vi "Delete Device.vi"(8 "Error In":errorcluster, 11 "Device In":T1) -> (0 "error out":errorcluster)   [LabVIEW 2012]
doc: "Deletes an OpenCLV device."
uses:
  Non-User VIs/Controls/Device ID.ctl
  Non-User VIs/Buffers/Buffer_states.ctl
  OpenCLV x64.lvlib
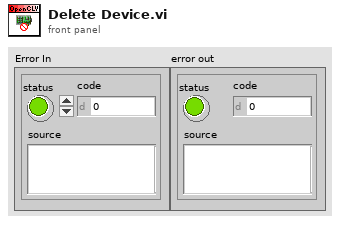
[diagram p1: front panel]
types:
  T1 = typedef "OpenCLV x64.lvlib/Device ID.ctl" = u64
  T2 = typedef "OpenCLV x64.lvlib/Buffer_states.ctl" = enum16{"Purge", "Remove", "Add"}
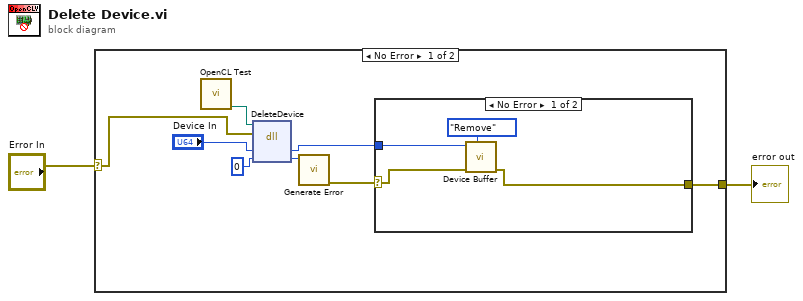
[diagram p0: block diagram]
diagram:
  n1 = case shown="No Error" "Error In" {
    selector: "Error In" -> [w3 w16]
    tunnel: [w10 w16] -> w2
    frame No Error {
      n2 = call "OpenCL Test.vi"() -> ("DLL To Use"=w4:path)  [unwired: 11 in]
      n3 = dll-call lib="C:/Users/bme-amcelroy-la/Desktop/OpenCLV/trunk/OpenCLV_x64_1.0/OpenCLV_x64.dll" fn="DeleteDevice"(path in=w4, error in=w3, "Device Handle"="Device In", "Error"=0) -> ("Device Handle"=w7:u64, "Error"=w6:i32)  [unwired: 2 in, 2 out]
      n4 = call "Generate Error.vi"("Error"=w6) -> ("error out"=w5:errorcluster)  [unwired: 10 in]
      n5 = case shown="No Error" w5 {
        selector: w5 -> [w11 w15]
        tunnel: [w12 w15] -> w10
        tunnel: w7 -> [w14 _]
        frame No Error {
          n6 = call "Device Buffer.vi"("States"=Buffer_states."Remove", "Error In"=w11, "Device"=w14) -> ("Error Out"=w12:errorcluster)  [unwired: 7 in, 1 out]
        }
        frame Error {
        }
      }
    }
    frame Error {
    }
  }
  "error out" <- w2
